vi "空调控制.vi"() -> ()   [LabVIEW 2016, in "环境动力监测库.lvlib" / "空调库.lvlib"]
uses:
  <vilib>/Utility/miscctls.llb/LVPointTypeDef.ctl
  <vilib>/Utility/config.llb/NI_LVConfig.lvlib
panel:
  in  "输入簇":T1={"监测项描述:输出"="", "连接方式"=enum."串口", "端口"="", "IP address:"="", "Port:"="", "站号"=19200, "传感器型号"="", "波特率"=19200, "data bits"=8, "停止位"=10, "奇偶校验"=0} {"停止位" items=["1.0"=10, "1.5"=15, "2.0"=20]; "奇偶校验" items=["None", "Odd", "Even", "Mark", "Space"]}
  in  "变更空调型号":bool
  out "布尔":bool
  # "空调监测"
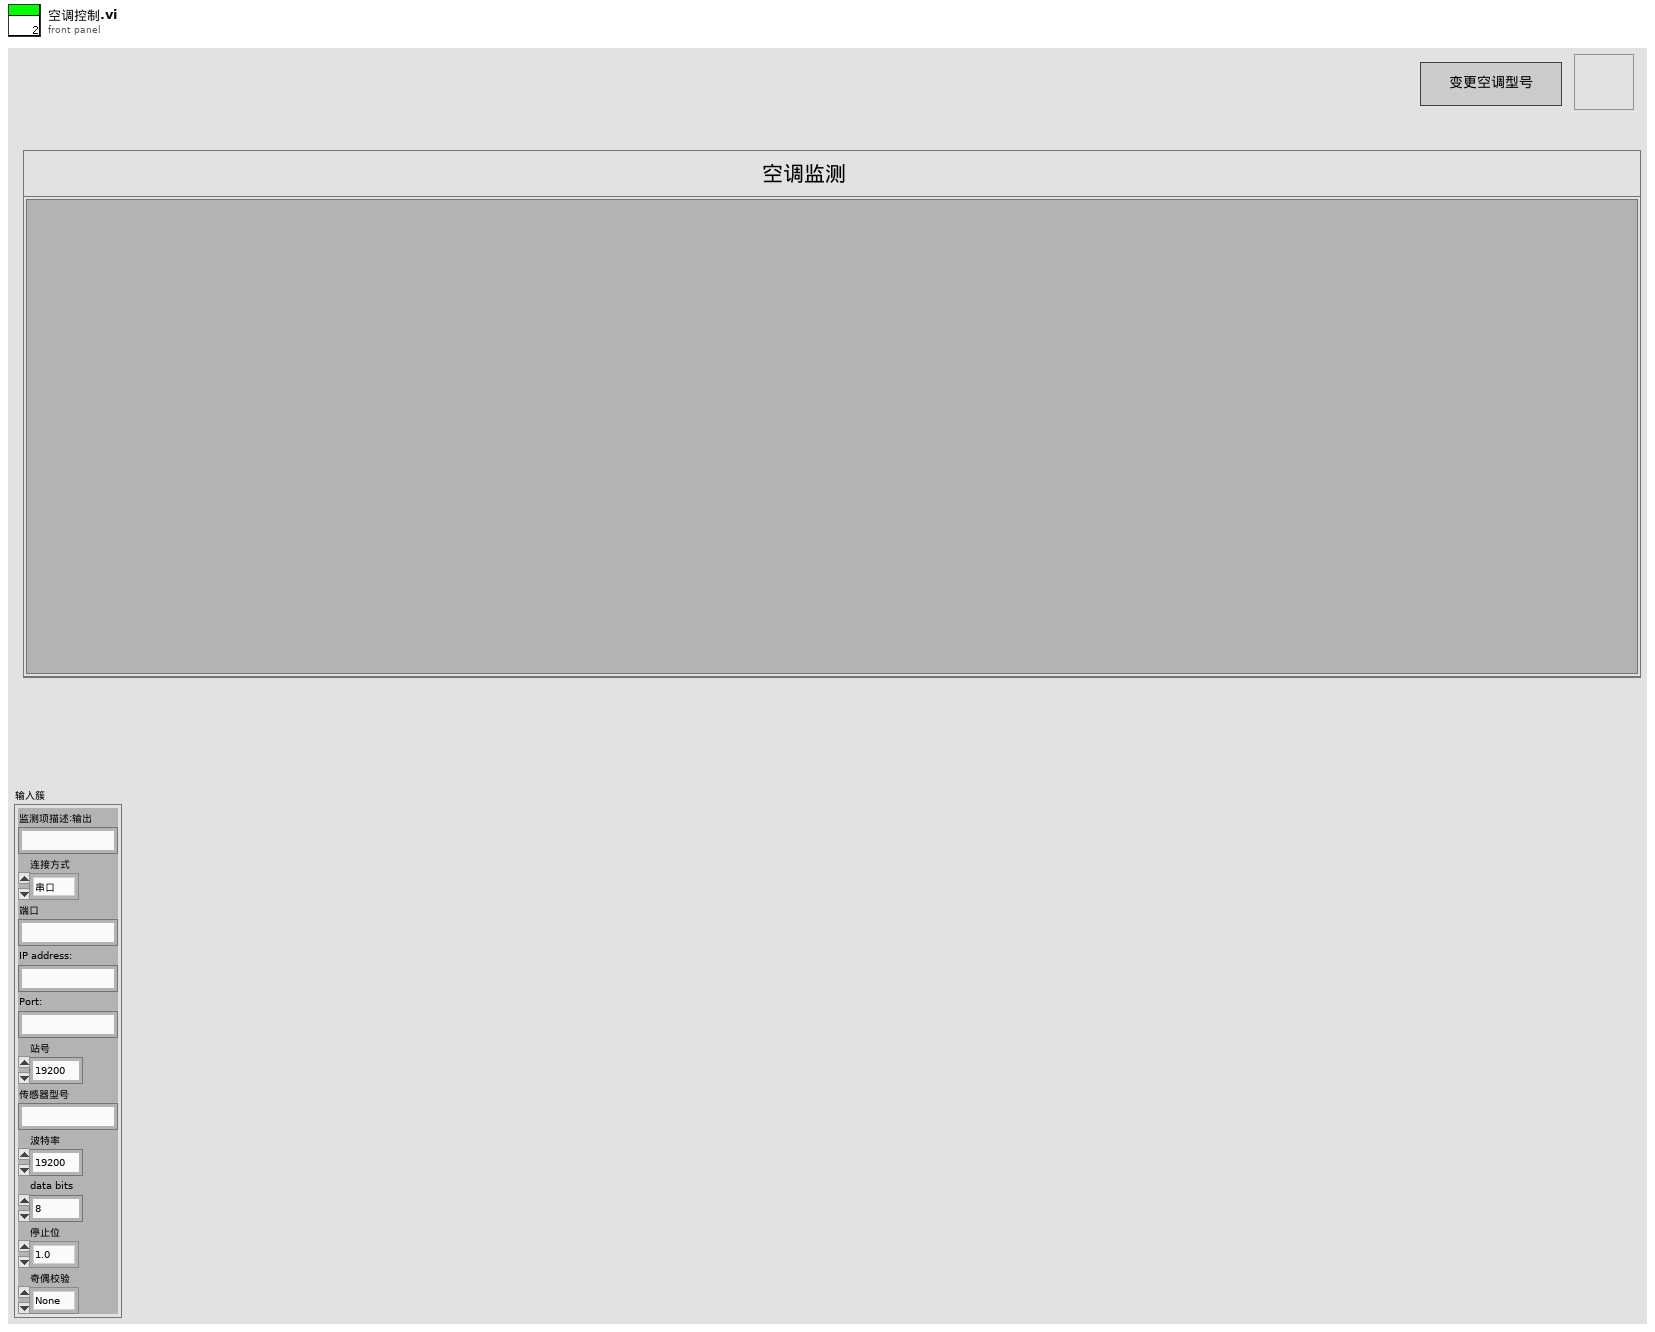
[diagram p1: front panel]
types:
  T1 = cluster{"监测项描述:输出":string, "连接方式":enum16{"串口", "TCP"}, "端口":string, "IP address:":string, "Port:":string, "站号":u64, "传感器型号":string, "波特率":u64, "data bits":u64, "停止位":u16, "奇偶校验":u16}
  T2 = cluster{"baud rate (bps)":u32, "stop bits":u16, "parity":u16, "flow control":u16, "timeout":u32, "retries":i32}
  T3 = typedef "NI_LVConfig.lvlib/Config Data RefNum.ctl" = refnum<k1>
  T4 = typedef "LVPointTypeDef.ctl" = cluster{"Horizontal":i16, "Vertical":i16}
  T5 = enum32{"Bad", "Idle", "Run top level", "Running"}
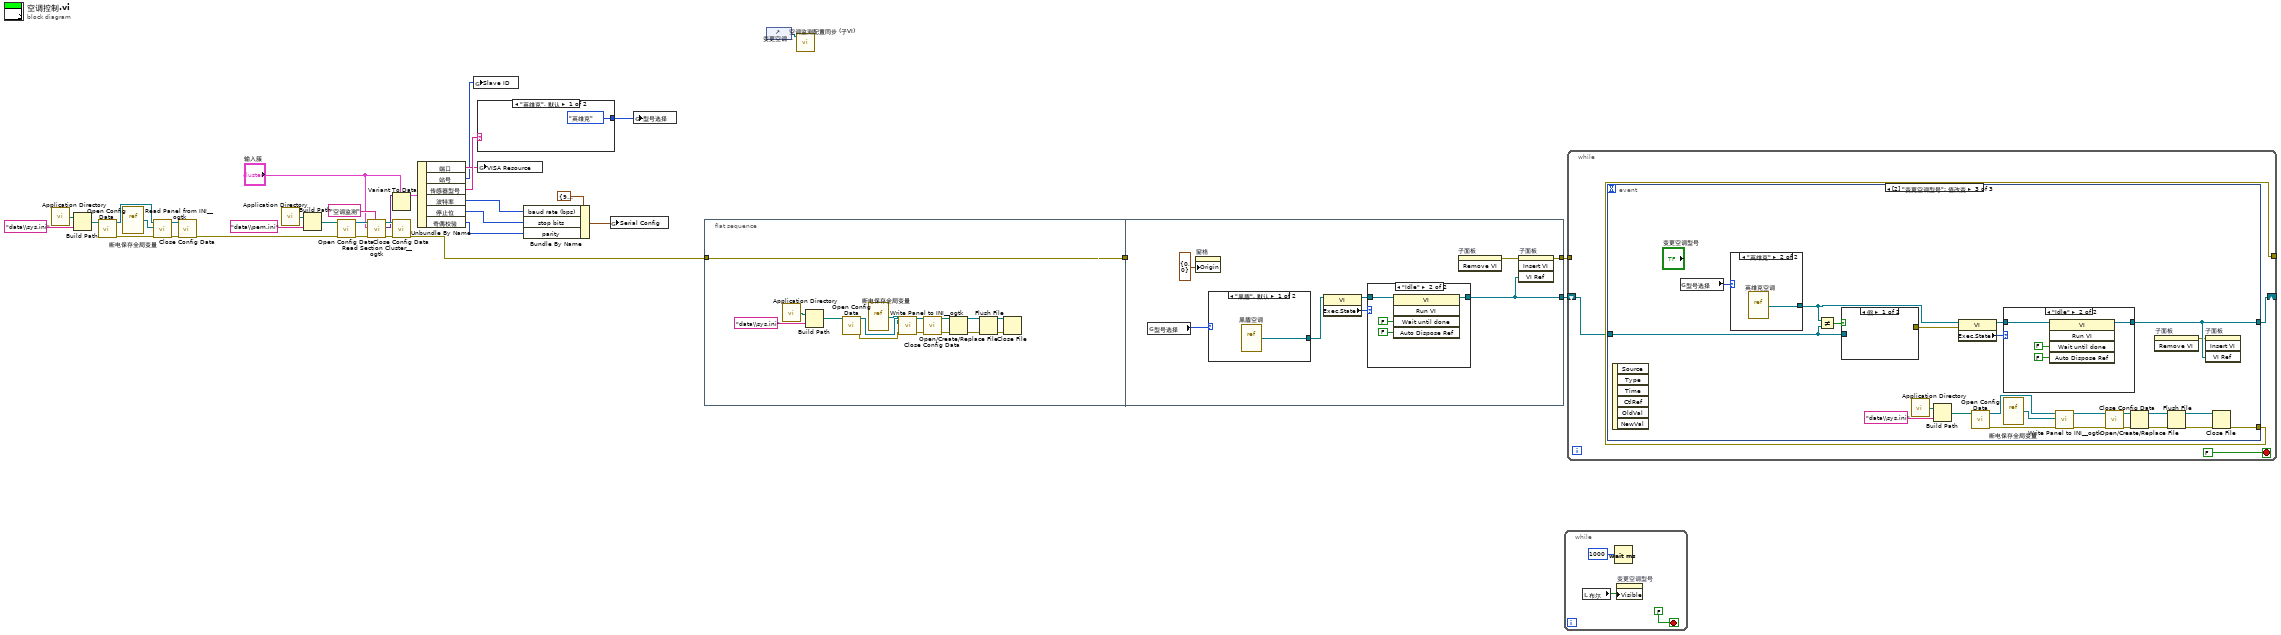
[diagram p0: block diagram]
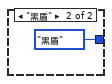
[diagram p2: hidden frame]
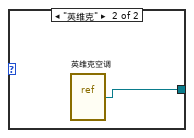
[diagram p3: hidden frame]
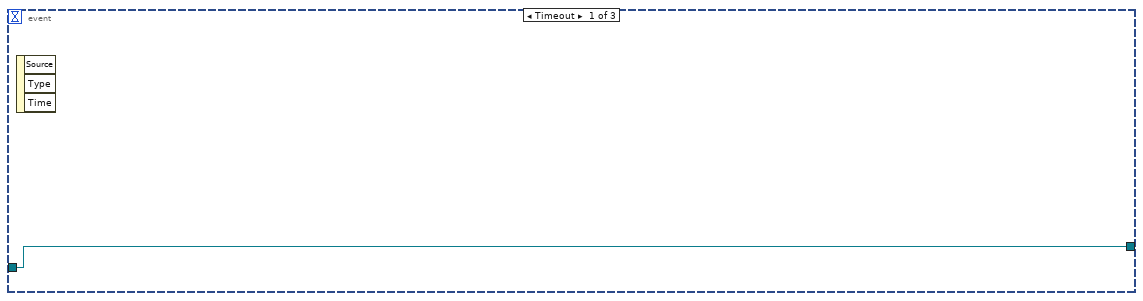
[diagram p5: hidden frame]
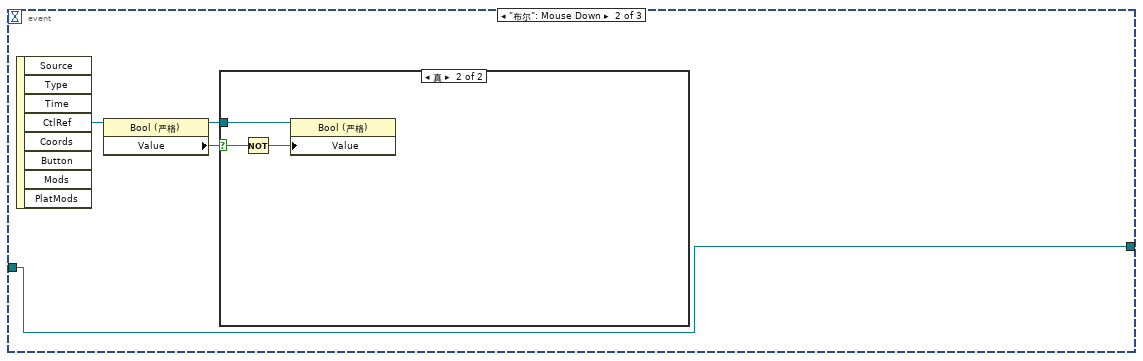
[diagram p6: hidden frame]
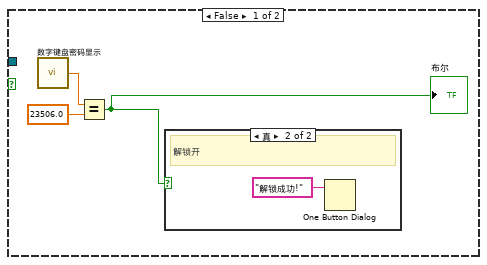
[diagram p7: hidden frame]
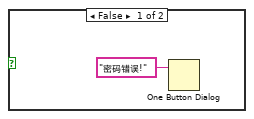
[diagram p8: hidden frame]
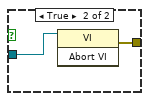
[diagram p9: hidden frame]
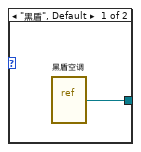
[diagram p10: hidden frame]
diagram:
  n1 = call <vilib>:"Application Directory.vi"() -> ("Application Directory"=w9:path)
  n2 = Build Path(base path=w9, name or relative path="data\\sys.ini" ("名称或相对路径")) -> (appended path=w7:path)
  n3 = call <vilib>:"Open Config Data.vi"("configuration file path"=w7) -> ("error out"=w3:errorcluster, "refnum"=w6:T3)  [unwired: 8 in, 1 out]
  n4 = vi-ref "断电保存全局变量.vi"() -> (w5:refnum<vi>)
  n5 = call <userlib>:"Read Panel from INI__ogtk.vi"("error in (no error)"=w3, "VI ref"=w5, "refnum"=w6) -> ("error out"=w2:errorcluster, "refnum out"=w4:T3)  [unwired: 7 in]
  n6 = call <vilib>:"Close Config Data.vi"("error in (no error)"=w2, "refnum"=w4) -> ("error out"=w1:errorcluster)  [unwired: 8 in, 1 out]
  n7 = call <vilib>:"Application Directory.vi"() -> ("Application Directory"=w30:path)
  n8 = Build Path(base path=w30, name or relative path="data\\pem.ini" ("名称或相对路径")) -> (appended path=w31:path)
  n9 = call <vilib>:"Open Config Data.vi"("error in (no error)"=w1, "configuration file path"=w31) -> ("error out"=w32:errorcluster, "refnum"=w33:T3)  [unwired: 7 in, 1 out]
  n10 = call <userlib>:"Read Section Cluster__ogtk.vi"("section (optional)"="空调监测", "error in (no error)"=w32, "Section Formatted Cluster Type"="输入簇", "refnum"=w33) -> ("error out"=w26:errorcluster, "Section Formatted Cluster"=w25:variant, "dup refnum"=w27:T3)  [unwired: 3 in, 2 out]
  n11 = Variant To Data(type="输入簇", Variant=w25) -> (data=w24:T1)  [unwired: 1 in, 1 out]
  n12 = call <vilib>:"Close Config Data.vi"("error in (no error)"=w26, "refnum"=w27) -> ("error out"=w18:errorcluster)  [unwired: 8 in, 1 out]
  n13 = Unbundle By Name(w24) -> ("端口"=w21:string, "站号"=w14:u64, "传感器型号"=w23:string, "波特率"=w13:u64, "停止位"=w12:u16, "奇偶校验"=w11:u16)
  n14 = global write "断电保存全局变量.vi" "Slave ID"(w14) -> ()
  n15 = case shown="\"英维克\", 默认" w23 {
    tunnel: [enum16{"黑盾", "英维克"}."英维克" ("型号选择") enum16{"黑盾", "英维克"}."黑盾" ("型号选择")] -> w22
    frame "英维克", Default {
    }
    frame "黑盾" {
    }
  }
  n16 = global write "断电保存全局变量.vi" "VISA Resource"(w21) -> ()
  n17 = Bundle By Name(cluster=T2 {"baud rate (bps)"=9600, "stop bits"=10, "parity"=0, "flow control"=0, "timeout"=1000, "retries"=1} ("Serial Config"), "baud rate (bps)"=w13, "stop bits"=w12, "parity"=w11) -> (w19:T2)
  n18 = global write "断电保存全局变量.vi" "Serial Config"(w19) -> ()
  n19 = global write "断电保存全局变量.vi" "型号选择"(w22) -> ()
  n20 = flat-sequence {
    tunnel: w18 -> [w51]
    tunnel: [w51] -> w17
    tunnel: [w54] -> w34
    tunnel: w17 -> [_]
    tunnel: [w53] -> w16
    frame #0 {
      n21 = call <vilib>:"Application Directory.vi"() -> ("Application Directory"=w49:path)
      n22 = Build Path(base path=w49, name or relative path="data\\sys.ini" ("名称或相对路径")) -> (appended path=w48:path)
      n23 = call <vilib>:"Open Config Data.vi"("configuration file path"=w48) -> ("error out"=w44:errorcluster, "refnum"=w47:T3)  [unwired: 8 in, 1 out]
      n24 = vi-ref "断电保存全局变量.vi"() -> (w46:refnum<vi>)
      n25 = call <userlib>:"Write Panel to INI__ogtk.vi"("error in (no error)"=w44, "VI ref"=w46, "refnum"=w47) -> ("error out"=w43:errorcluster, "refnum out"=w45:T3)  [unwired: 7 in]
      n26 = call <vilib>:"Close Config Data.vi"("error in (no error)"=w43, "refnum"=w45) -> ("error out"=w38:errorcluster, "file path"=w37:path)  [unwired: 8 in]
      n27 = Open/Create/Replace File(file path (use dialog)=w37, error in=w38) -> (refnum out=w41:refnum<file>, error out=w42:errorcluster)  [unwired: 4 in, 1 out]
      n28 = Flush File(refnum=w41, error in=w42) -> (refnum out=w40:refnum<file>, error out=w39:errorcluster)
      n29 = Close File(refnum=w40, error in=w39) -> ()  [unwired: 2 out]
    }
    frame #1 {
      n30 = global read "断电保存全局变量.vi" "型号选择"() -> (w56:enum16{"黑盾", "英维克"})
      n31 = property on="窗格" class="Pane"("Origin"=T4 {"Horizontal"=0, "Vertical"=0} ("原点")) -> ()  [unwired: 2 in, 2 out]
      n32 = case shown="\"黑盾\", 默认" w56 {
        tunnel: [w60 w61] -> w55
        frame "黑盾", Default {
          n33 = vi-ref "黑盾空调.vi"() -> (w60:refnum<vi>)
        }
        frame "英维克" {
          n34 = vi-ref "英维克空调.vi"() -> (w61:refnum<vi>)
        }
      }
      n35 = property class="VI"(reference=w55) -> (reference out=w58:refnum<vi>, "Exec.State"=w59:T5)  [unwired: 1 in, 1 out]
      n36 = case shown="\"Idle\"" w59 {
        tunnel: w58 -> [w62 w64]
        tunnel: [w62 w63] -> w53
        frame "Bad", Default {
        }
        frame "Idle" {
          n37 = invoke class="VI" method="Run VI"(reference=w64, "Wait until done"=FALSE ("结束前等待"), "Auto Dispose Ref"=FALSE ("自动销毁引用")) -> (reference out=w63:refnum<vi>)  [unwired: 2 in, 4 out]
        }
      }
      n38 = invoke on="子面板" class="SubPnl" method="Remove VI"() -> (error out=w57:errorcluster)  [unwired: 3 in, 2 out]
      n39 = invoke on="子面板" class="SubPnl" method="Insert VI"(error in=w57, "VI Ref"=w53) -> (error out=w54:errorcluster)  [unwired: 2 in, 3 out]
    }
  }
  n40 = control-ref of="变更空调型号"() -> (w10:refnum<vi>)
  n41 = call "空调监测配置同步 (子VI).vi"("Boolean输入"=w10) -> ()  [unwired: 11 in]
  n42 = while {
    stop <- FALSE stop-if-true
    n43 = local read "布尔"() -> (w68:bool)
    n44 = Wait (ms)(milliseconds to wait=u32 1000 ("等待时间（毫秒）")) -> ()  [unwired: 1 out]
    n45 = property on="变更空调型号" class="Bool (严格)"("Visible"=w68) -> ()  [unwired: 2 in, 2 out]
  }
  n46 = while {
    tunnel: w34 -> [_]
    tunnel: [w73] -> _
    shift-right: [w72] -> _
    shift-left: w16 -> [w71]
    stop <- FALSE stop-if-true
    n47 = event shown="[2] \"变更空调型号\": 值改变" {
      selector: _ -> [_ _ _]
      dyn-events: _ -> [_ _ _]
      timeout: _ -> [_ _ _]
      tunnel: [_ _ w110] -> w73
      tunnel: [w74 w75 w109] -> w72
      tunnel: w71 -> [w74 w75 w89]
      event Timeout {
        n48 = event-data() -> ()  [unwired: 1 in, 3 out]
      }
      event "布尔": Mouse Down {
        n49 = event-data() -> ("CtlRef"=w78:refnum<vi>)  [unwired: 1 in, 7 out]
        n50 = property class="Bool (严格)"(reference=w78) -> (reference out=w76:refnum<vi>, "Value"=w77:bool)  [unwired: 1 in, 1 out]
        n51 = case shown="真" w77 {
          selector: w77 -> [_ w86]
          tunnel: w76 -> [_ w85]
          frame False {
            n52 = call "数字键盘密码显示.vi"() -> ("NewNumber"=w81:sgl)  [unwired: 1 in]
            n53 = Equal?(x=w81, y=sgl 23506.0) -> (x = y?=w79:bool)
            "布尔" <- w79
            n54 = case shown="真" w79 {
              frame False {
                n55 = One Button Dialog(message="密码错误!" ("消息")) -> ()  [unwired: 1 in, 1 out]
              }
              frame True {
                # "解锁开"
                n56 = One Button Dialog(message="解锁成功!" ("消息")) -> ()  [unwired: 1 in, 1 out]
              }
            }
          }
          frame True {
            n57 = Not(x=w86) -> (.not. x?=w84:bool)
            n58 = property class="Bool (严格)"(reference=w85, "Value"=w84) -> ()  [unwired: 1 in, 2 out]
          }
        }
      }
      event "变更空调型号": Value Change {
        n59 = event-data() -> ()  [unwired: 1 in, 6 out]
        n60 = global read "断电保存全局变量.vi" "型号选择"() -> (w90:enum16{"黑盾", "英维克"})
        n61 = case shown="\"英维克\"" w90 {
          tunnel: [w113 w114] -> w88
          frame "黑盾", Default {
            n62 = vi-ref "黑盾空调.vi"() -> (w113:refnum<vi>)
          }
          frame "英维克" {
            n63 = vi-ref "英维克空调.vi"() -> (w114:refnum<vi>)
          }
        }
        n64 = Not Equal?(x=w88, y=w89) -> (x != y?=w87:bool)
        n65 = case shown="假" w87 {
          tunnel: w89 -> [_ w112]
          tunnel: [_ w111] -> w91
          frame False {
          }
          frame True {
            n66 = invoke class="VI" method="Abort VI"(reference=w112) -> (error out=w111:errorcluster)  [unwired: 2 in, 2 out]
          }
        }
        n67 = call <vilib>:"Application Directory.vi"() -> ("Application Directory"=w104:path)
        n68 = Build Path(base path=w104, name or relative path="data\\sys.ini" ("名称或相对路径")) -> (appended path=w103:path)
        n69 = property class="VI"(reference=w88, error in=w91) -> (reference out=w107:refnum<vi>, "Exec.State"=w108:T5)  [unwired: 1 out]
        n70 = call <vilib>:"Open Config Data.vi"("configuration file path"=w103) -> ("error out"=w99:errorcluster, "refnum"=w102:T3)  [unwired: 8 in, 1 out]
        n71 = case shown="\"Idle\"" w108 {
          tunnel: w107 -> [w115 w117]
          tunnel: [w115 w116] -> w109
          frame "Bad", Default {
          }
          frame "Idle" {
            n72 = invoke class="VI" method="Run VI"(reference=w117, "Wait until done"=FALSE ("结束前等待"), "Auto Dispose Ref"=FALSE ("自动销毁引用")) -> (reference out=w116:refnum<vi>)  [unwired: 2 in, 4 out]
          }
        }
        n73 = vi-ref "断电保存全局变量.vi"() -> (w101:refnum<vi>)
        n74 = call <userlib>:"Write Panel to INI__ogtk.vi"("error in (no error)"=w99, "VI ref"=w101, "refnum"=w102) -> ("error out"=w98:errorcluster, "refnum out"=w100:T3)  [unwired: 7 in]
        n75 = call <vilib>:"Close Config Data.vi"("error in (no error)"=w98, "refnum"=w100) -> ("error out"=w93:errorcluster, "file path"=w92:path)  [unwired: 8 in]
        n76 = Open/Create/Replace File(file path (use dialog)=w92, error in=w93) -> (refnum out=w96:refnum<file>, error out=w97:errorcluster)  [unwired: 4 in, 1 out]
        n77 = invoke on="子面板" class="SubPnl" method="Remove VI"() -> (error out=w106:errorcluster)  [unwired: 3 in, 2 out]
        n78 = Flush File(refnum=w96, error in=w97) -> (refnum out=w95:refnum<file>, error out=w94:errorcluster)
        n79 = invoke on="子面板" class="SubPnl" method="Insert VI"(error in=w106, "VI Ref"=w109) -> ()  [unwired: 2 in, 4 out]
        n80 = Close File(refnum=w95, error in=w94) -> (error out=w110:errorcluster)  [unwired: 1 out]
      }
    }
  }
